vi "Actor Core.vi"(8 "error in":errorcluster, 11 "RootModelPublishesUnthrottled in":refnum<class "ModelPublishesIndexA.lvclass">) -> (0 "error out":errorcluster, 3 "Actor out":refnum<class "Actor.lvclass">)   [LabVIEW 2020, in "BenchmarkObservationRate.lvlib" / "ModelPublishesIndexA.lvclass"]
doc: "(<B>Filename</B>: Actor Framework.lvlib:Actor.lvclass:Actor Core.vi)\n\nReceives messages to the actor, reacts to them, and initiates any error handling that may shut the actor down.\n\nDescendant classes may override this VI to append parallel tasks for the actor to complete while it handles messages. Overrides use the Call Parent Method node."
uses:
  ModelPublishesIndexA.lvclass
  ModelPublishesIndexA.lvclass/ModelPublishesIndexA.ctl
  <vilib>/ActorFramework/Actor/Actor.lvclass
  Source/IModel/IModel/IModel.lvclass
  C:/Git/mva-core/Source/IModel/IModel/IModel.lvclass
  C:/Git/mva-core/Source/IObserver/IObserver/IObserver.lvclass
  C:/Program Files (x86)/National Instruments/LabVIEW 2020/vi.lib/ActorFramework/Actor/Actor.lvclass
  C:/Git/mva-core/Test/BechmarkObservationRate/Doubles/RootModelPublishesUnthrottled/ModelPublishesIndexA.lvclass
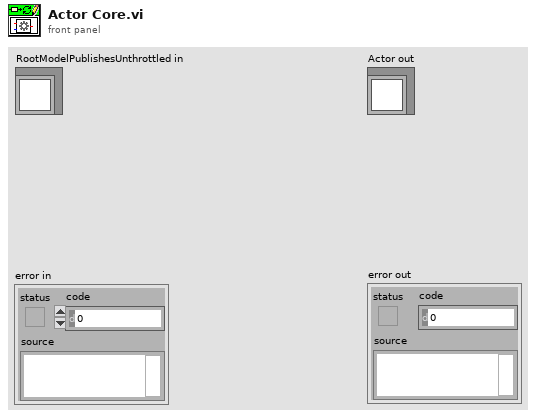
[diagram p1: front panel]
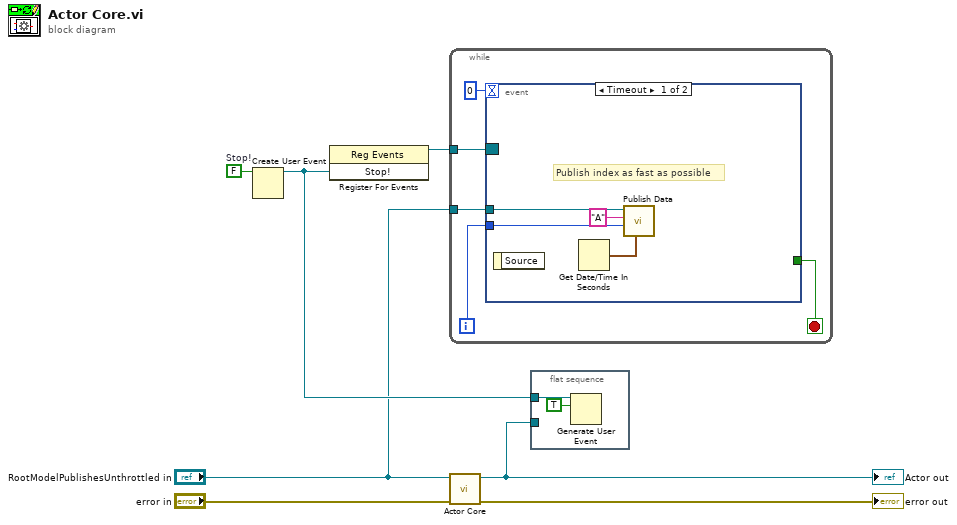
[diagram p0: block diagram]
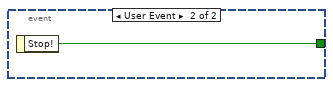
[diagram p2: hidden frame]
diagram:
  w3 = FALSE  # Stop!
  n1 = Create User Event(user event datatype=w3) -> (user event=w5:refnum<user-event>)  [unwired: 1 in, 1 out]
  n2 = register-events(w5) -> (reference out=w2:refnum<event-registration>)  [unwired: 2 in, 1 out]
  n3 = while {
    tunnel: w2 -> [w11]
    tunnel: "RootModelPublishesUnthrottled in" -> [w10]
    i -> [w9]
    stop <- w8 stop-if-true
    n4 = event shown="[0] Timeout" {
      selector: w11 -> [_ _]
      dyn-events: _ -> [_ _]
      timeout: 0 -> [_ _]
      tunnel: w10 -> [w16 _]
      tunnel: w9 -> [w14 _]
      tunnel: [_ w17] -> w8
      event Timeout {
        # "Publish index as fast as possible"
        n5 = event-data() -> ()  [unwired: 1 in, 1 out]
        n6 = Get Date/Time In Seconds() -> (seconds since 1Jan1904=w13:timestamp)
        n7 = call "Publish Data.vi"("Publish Time (Use Current Time)"=w13, "Data to Publish"=w14, "Datum Name"="A", "IModel in"=w16) -> ()  [unwired: 6 in, 2 out]
      }
      event User Event {
        n8 = event-data() -> ("Stop!"=w17:bool)  [unwired: 1 in]
      }
    }
  }
  n9 = call-parent "Actor Core.vi"("error in"="error in", "Actor in"="RootModelPublishesUnthrottled in") -> ("error out"=→"error out":errorcluster, "Actor out"=w4:refnum<class "Actor.lvclass">)  [unwired: 8 in]
  "Actor out" <- w4
  n10 = flat-sequence {
    tunnel: w5 -> [w19]
    tunnel: w4 -> [_]
    frame #0 {
      n11 = Generate User Event(user event=w19, event data cluster=TRUE ("event data")) -> ()  [unwired: 2 in, 2 out]
    }
  }
